vi "Update Color Index Array.vi"(4 "Y Dimension":i32, 6 "X Dimension":i32, 7 "Ribbon Mode":enum16{"Row", "Column"}(ring), 11 "Color Index Array In":i32[](array[numeric])) -> (3 "Color Index Array Out":i32[](array[numeric]))   [LabVIEW 2020, in "3D Ribbon.lvclass"]
uses:
  <vilib>/Math Plots/3D Math Plots/3D Ribbon/3D Ribbon/3D Ribbon.lvclass
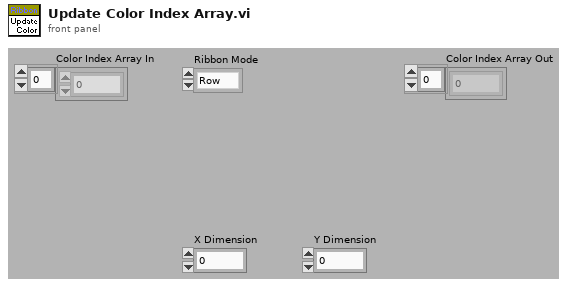
[diagram p1: front panel]
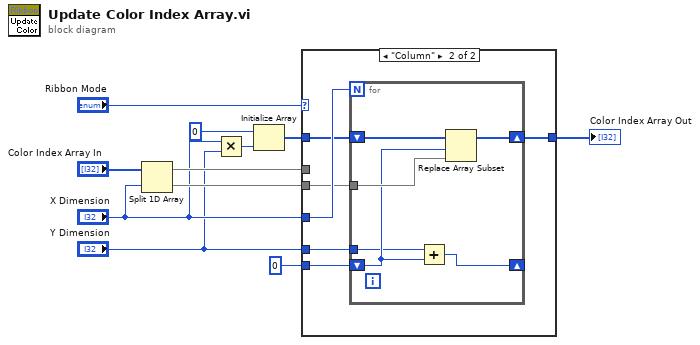
[diagram p0: block diagram]
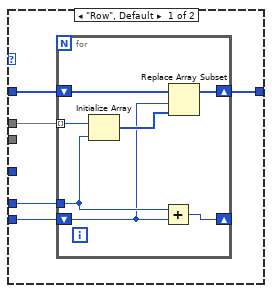
[diagram p2: hidden frame]
diagram:
  n1 = Split 1D Array(array="Color Index Array In", index="X Dimension") -> (first subarray=w9:i32[], second subarray=w8:i32[])
  n2 = Multiply(x="X Dimension", y="Y Dimension") -> (x*y=w6:i32)
  n3 = Initialize Array(0, w6) -> (w2:i32[])
  n4 = case shown="\"Column\"" "Ribbon Mode" {
    tunnel: "Y Dimension" -> [w14 w24]
    tunnel: w9 -> [w15 _]
    tunnel: w8 -> [_ w25]
    tunnel: "X Dimension" -> [_ w28]
    tunnel: [w16 w29] -> w7
    tunnel: w2 -> [w13 w27]
    tunnel: 0 -> [w12 w26]
    frame "Row", Default {
      n5 = for {
        tunnel: w15 -> [w21] mode=indexing
        shift-right: [w23] -> w16
        shift-left: w13 -> [w22]
        tunnel: w14 -> [w19]
        shift-right: [w18] -> _
        shift-left: w12 -> [w17]
        n6 = Initialize Array(w21, w19) -> (w20:i32[])
        n7 = Add(x=w19, y=w17) -> (x+y=w18:i32)
        n8 = Replace Array Subset(array=w22, new element=w20, index=w17) -> (w23:i32[])
      }
    }
    frame "Column" {
      n9 = for {
        N: w28 -> [_]
        tunnel: w25 -> [w33]
        shift-right: [w35] -> w29
        shift-left: w27 -> [w34]
        shift-right: [w31] -> _
        shift-left: w26 -> [w32]
        tunnel: w24 -> [w30]
        n10 = Add(x=w30, y=w32) -> (x+y=w31:i32)
        n11 = Replace Array Subset(array=w34, new element=w33, index=w32) -> (w35:i32[])
      }
    }
  }
  "Color Index Array Out" <- w7
